vi "Keithley 3390 Modulation.vi"() -> ()   [LabVIEW 2017]
doc: "This example demonstraights how to configure the function generator to output a modulated signal."
uses:
  Keithley 3390.lvlib
  Public/Configure/Configure Waveform (Sine).vi
  Public/Configure/Configure Modulation (Amplitude).vi
panel:
  in  "Modulation Depth (100 %)":i32=100 min=0 max=120
  in  "Modulation Frequency (100 Hz)":dbl=100.0
  in  "Modulation Waveform (Sine)":T1(ring)
  in  "AM Source (Internal)":enum16{"Internal", "External"}(ring)
  in  "Frequency (1000 Hz)":dbl=1000.0
  in  "DC Offset (0.00 V)":dbl
  in  "Amplitude (1.0 Vpp)":dbl=1.0
  in  "VISA resource name":refnum<visa-resource-name>
  # "(c) 2008 Keithley Instruments, Inc.  ALL RIGHTS RESERVED."
  # "Carrier Waveform Settings"
  # "Modulating Waveform Settings"
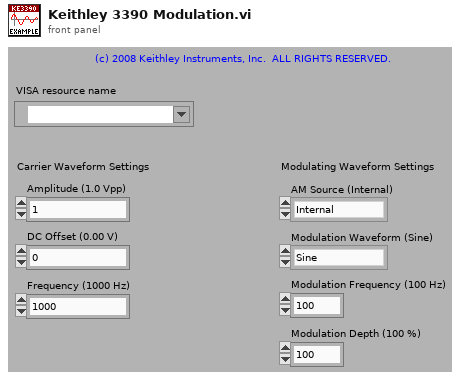
[diagram p1: front panel]
types:
  T1 = enum16{"Sine", "Square", "Ramp", "Negative Ramp", "Triangle", "Noise", "Arbitrary"}
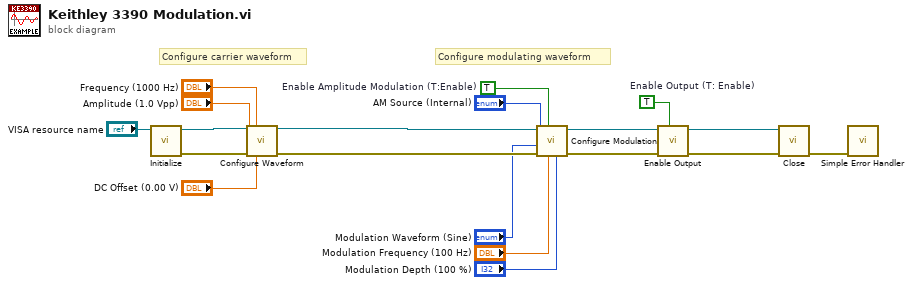
[diagram p0: block diagram]
diagram:
  w6 = TRUE  # Enable Amplitude Modulation (T:Enable)
  w11 = TRUE  # Enable Output (T: Enable)
  # "Configure modulating waveform"
  # "Configure carrier waveform"
  n1 = call "Initialize.vi"("VISA resource name"="VISA resource name") -> ("error out"=w19:errorcluster, "VISA resource name out"=w17:refnum<visa-resource-name>)  [unwired: 9 in]
  n2 = call-poly "Configure Waveform.vi"("VISA resource name"=w17, "Frequency (1000 Hz)"="Frequency (1000 Hz)", "Amplitude (1.0 Vpp)"="Amplitude (1.0 Vpp)", "error in (no error)"=w19, "DC Offset (0.00 V)"="DC Offset (0.00 V)") -> ("VISA resource name out"=w16:refnum<visa-resource-name>, "error out"=w18:errorcluster)  [unwired: 9 in]
  n3 = call-poly "Configure Modulation.vi"("Modulation Depth (100 %)"="Modulation Depth (100 %)", "Modulation Frequency (100 Hz)"="Modulation Frequency (100 Hz)", "Enable Amplitude Modulation (T:Enable)"=w6, "error in (no error)"=w18, "Modulation Waveform (Sine)"="Modulation Waveform (Sine)", "AM Source (Internal)"="AM Source (Internal)", "VISA resource name"=w16) -> ("error out"=w14:errorcluster, "VISA resource name out"=w10:refnum<visa-resource-name>)  [unwired: 3 in]
  n4 = call "Enable Output.vi"("Enable Output (T: Enable)"=w11, "error in (no error)"=w14, "VISA resource name"=w10) -> ("error out"=w13:errorcluster, "VISA resource name out"=w12:refnum<visa-resource-name>)  [unwired: 7 in]
  n5 = call "Close.vi"("error in (no error)"=w13, "VISA resource name"=w12) -> ("error out"=w1:errorcluster)  [unwired: 9 in]
  n6 = call <vilib>:"Simple Error Handler.vi"("error in (no error)"=w1) -> ()  [unwired: 4 in, 5 out]
